vi "Constant - Wait Time (ms).vi"() -> (3 "milliseconds to wait":u32=100)   [LabVIEW 2020]
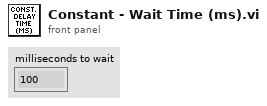
[diagram p1: front panel]
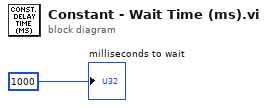
[diagram p0: block diagram]
diagram:
  "milliseconds to wait" <- u32 1000 ("milliseconds to wait")
